vi "NavX Zero Heading.vi"(8 "error in":errorcluster) -> (0 "error out":errorcluster)   [LabVIEW 2014]
uses:
  Global Objects.vi
  navX Library v2/navX Library v2.lvlib
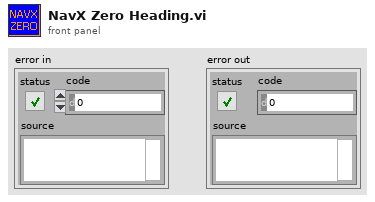
[diagram p1: front panel]
types:
  T1 = typedef "NaxX Info.ctl" = cluster{"navX Device":T2, "Previous Heading":dbl, "Zeroed Heading":dbl}
  T2 = typedef "navX Library v2.lvlib/Z900_navX_DeviceTypeDef.ctl" = cluster{"Interface":cluster{"Protocol":T3, "Update Rate (4Hz-60Hz)":u8, "navX Open TypeDef":variant}, "Notify Packet":refnum<notifier>, "Loop VI Refnum":refnum<vi>, "Ready to Close Occurrence Refnum":refnum<k4>}
  T3 = typedef "navX Library v2.lvlib/Z900_navX_ProtocolTypeDef.ctl" = enum16{"SERIAL", "I2C", "SPI"}
  T4 = cluster{"Yaw":dbl, "Roll":dbl, "Pitch":dbl, "Heading":dbl, "Fused Heading":dbl}
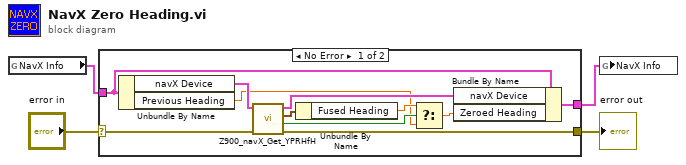
[diagram p0: block diagram]
diagram:
  n1 = global read "Global Objects.vi" "NavX Info"() -> (w2:T1)
  n2 = case shown="No Error" "error in" {
    selector: "error in" -> [w12 w17]
    tunnel: [w11 w17] -> w3
    tunnel: w2 -> [w14 w16]
    tunnel: [w15 w16] -> w1
    frame No Error {
      n3 = Unbundle By Name(w14) -> ("navX Device"=w13:T2, "Previous Heading"=w6:dbl)
      n4 = call "Z900_navX_Get_YPRHfH.vi"("error in (no error)"=w12, "navX Device"=w13) -> ("error out"=w11:errorcluster, "Connected"=w10:bool, "YRPHfH"=w9:T4, "navX Device"=w8:T2)  [unwired: 6 in]
      n5 = Unbundle By Name(w9) -> ("Fused Heading"=w7:dbl)
      n6 = Select(t=w7, s=w10, f=w6) -> (s? t:f=w5:dbl)
      n7 = Bundle By Name(cluster=w14, "navX Device"=w8, "Zeroed Heading"=w5) -> (w15:T1)
    }
    frame Error {
    }
  }
  "error out" <- w3
  n8 = global write "Global Objects.vi" "NavX Info"(w1) -> ()
